vi "monitor_old.vi"() -> ()   [LabVIEW 2010]
uses:
  <vilib>/Instr/_visa.llb/VISA Configure Serial Port (Instr).vi
panel:
  out "start time":timestamp
  in  "Boolean 6":bool
  in  "Log file":path=path "C:/write-read example.txt"
  in  "Boolean 5":bool
  in  "Log file":path=path "C:/write-read example.txt"
  in  "Boolean 4":bool
  in  "Log file":path=path "C:/write-read example.txt"
  in  "Boolean 3":bool
  in  "Log file":path=path "C:/write-read example.txt"
  in  "Boolean 2":bool
  in  "Log file":path=path "C:/write-read example.txt"
  in  "Boolean":bool
  in  "Log file":path=path "C:/write-read example.txt"
  out "Power":dbl format="%.2g"
  out "Power":dbl format="%.2g"
  out "Power":dbl format="%.2g"
  out "Power":dbl format="%.2g"
  out "Power":dbl format="%.2g"
  out "Power":dbl format="%.2g"
  out "readPower":string=">\\s$R153\\?\\r\\n"
  in  "Connect all":bool
  out "Voltage":dbl format="%.2g"
  out "Current":dbl format="%.2g"
  out "Regulator":dbl format="%.2g"
  out "Extra sensor":dbl format="%.2g"
  out "Cold plate":dbl format="%.2g"
  out "Set point":dbl format="%.2g"
  out "Main sensor":dbl format="%.2g"
  out "Voltage":dbl format="%.2g"
  out "Current":dbl format="%.2g"
  out "Regulator":dbl format="%.2g"
  out "Extra sensor":dbl format="%.2g"
  out "Cold plate":dbl format="%.2g"
  out "Set point":dbl format="%.2g"
  out "Sensor":dbl format="%.2g"
  out "Voltage":dbl format="%.2g"
  out "Current":dbl format="%.2g"
  out "Regulator":dbl format="%.2g"
  out "Extra sensor":dbl format="%.2g"
  out "Cold plate":dbl format="%.2g"
  out "Set point":dbl format="%.2g"
  out "Main sensor":dbl format="%.2g"
  out "Voltage":dbl format="%.2g"
  out "Current":dbl format="%.2g"
  out "Regulator":dbl format="%.2g"
  out "Extra sensor":dbl format="%.2g"
  out "Cold plate":dbl format="%.2g"
  out "Set point":dbl format="%.2g"
  out "Sensor":dbl format="%.2g"
  out "Voltage":dbl format="%.2g"
  out "Current":dbl format="%.2g"
  out "Regulator":dbl format="%.2g"
  out "Extra sensor":dbl format="%.2g"
  out "Cold plate":dbl format="%.2g"
  out "Set point":dbl format="%.2g"
  out "Main sensor":dbl format="%.2g"
  out "readI":string=">\\s$R101\\?\\r\\n"
  out "readV":string=">\\s$R101\\?\\r\\n"
  out "readT4":string=">\\s$R101\\?\\r\\n"
  out "Voltage":dbl format="%.2g"
  out "Current":dbl format="%.2g"
  out "Regulator":dbl format="%.2g"
  out "readT3":string=">\\s$R101\\?\\r\\n"
  out "Extra sensor":dbl format="%.2g"
  out "Cold plate":dbl format="%.2g"
  out "Set point":dbl format="%.2g"
  out "readT2":string=">\\s$R101\\?\\r\\n"
  out "readT1":string=">\\s$R100\\?\\r\\n"
  out "readSetPoint":string="$R0\\?\\r\\n"
  out "Main sensor":dbl format="%.2g"
  in  "Port":refnum<visa-resource-name>="COM7"
  in  "Port":refnum<visa-resource-name>="COM6"
  in  "Port":refnum<visa-resource-name>="COM11"
  in  "Port":refnum<visa-resource-name>="COM10"
  in  "Port":refnum<visa-resource-name>="COM9"
  in  "Port":refnum<visa-resource-name>="COM8"
  in  "stop":bool
  # "Top S"
  # "Top N"
  # "Temeprature"
  # "Temeprature"
  # "Bottom S"
  # "Bottom N"
  # "Temeprature"
  # "Temeprature"
  # "Front S"
  # "Front N"
  # "Temeprature"
  # "Temeprature"
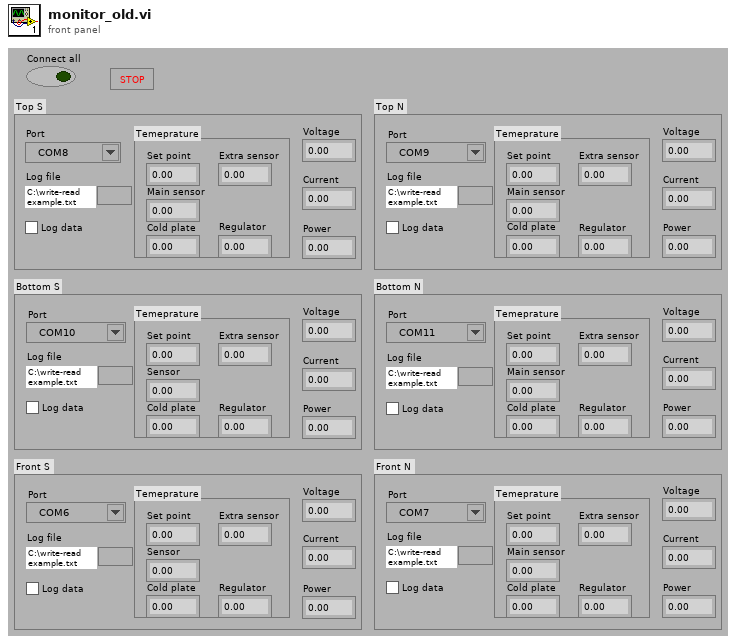
[diagram p1: front panel]
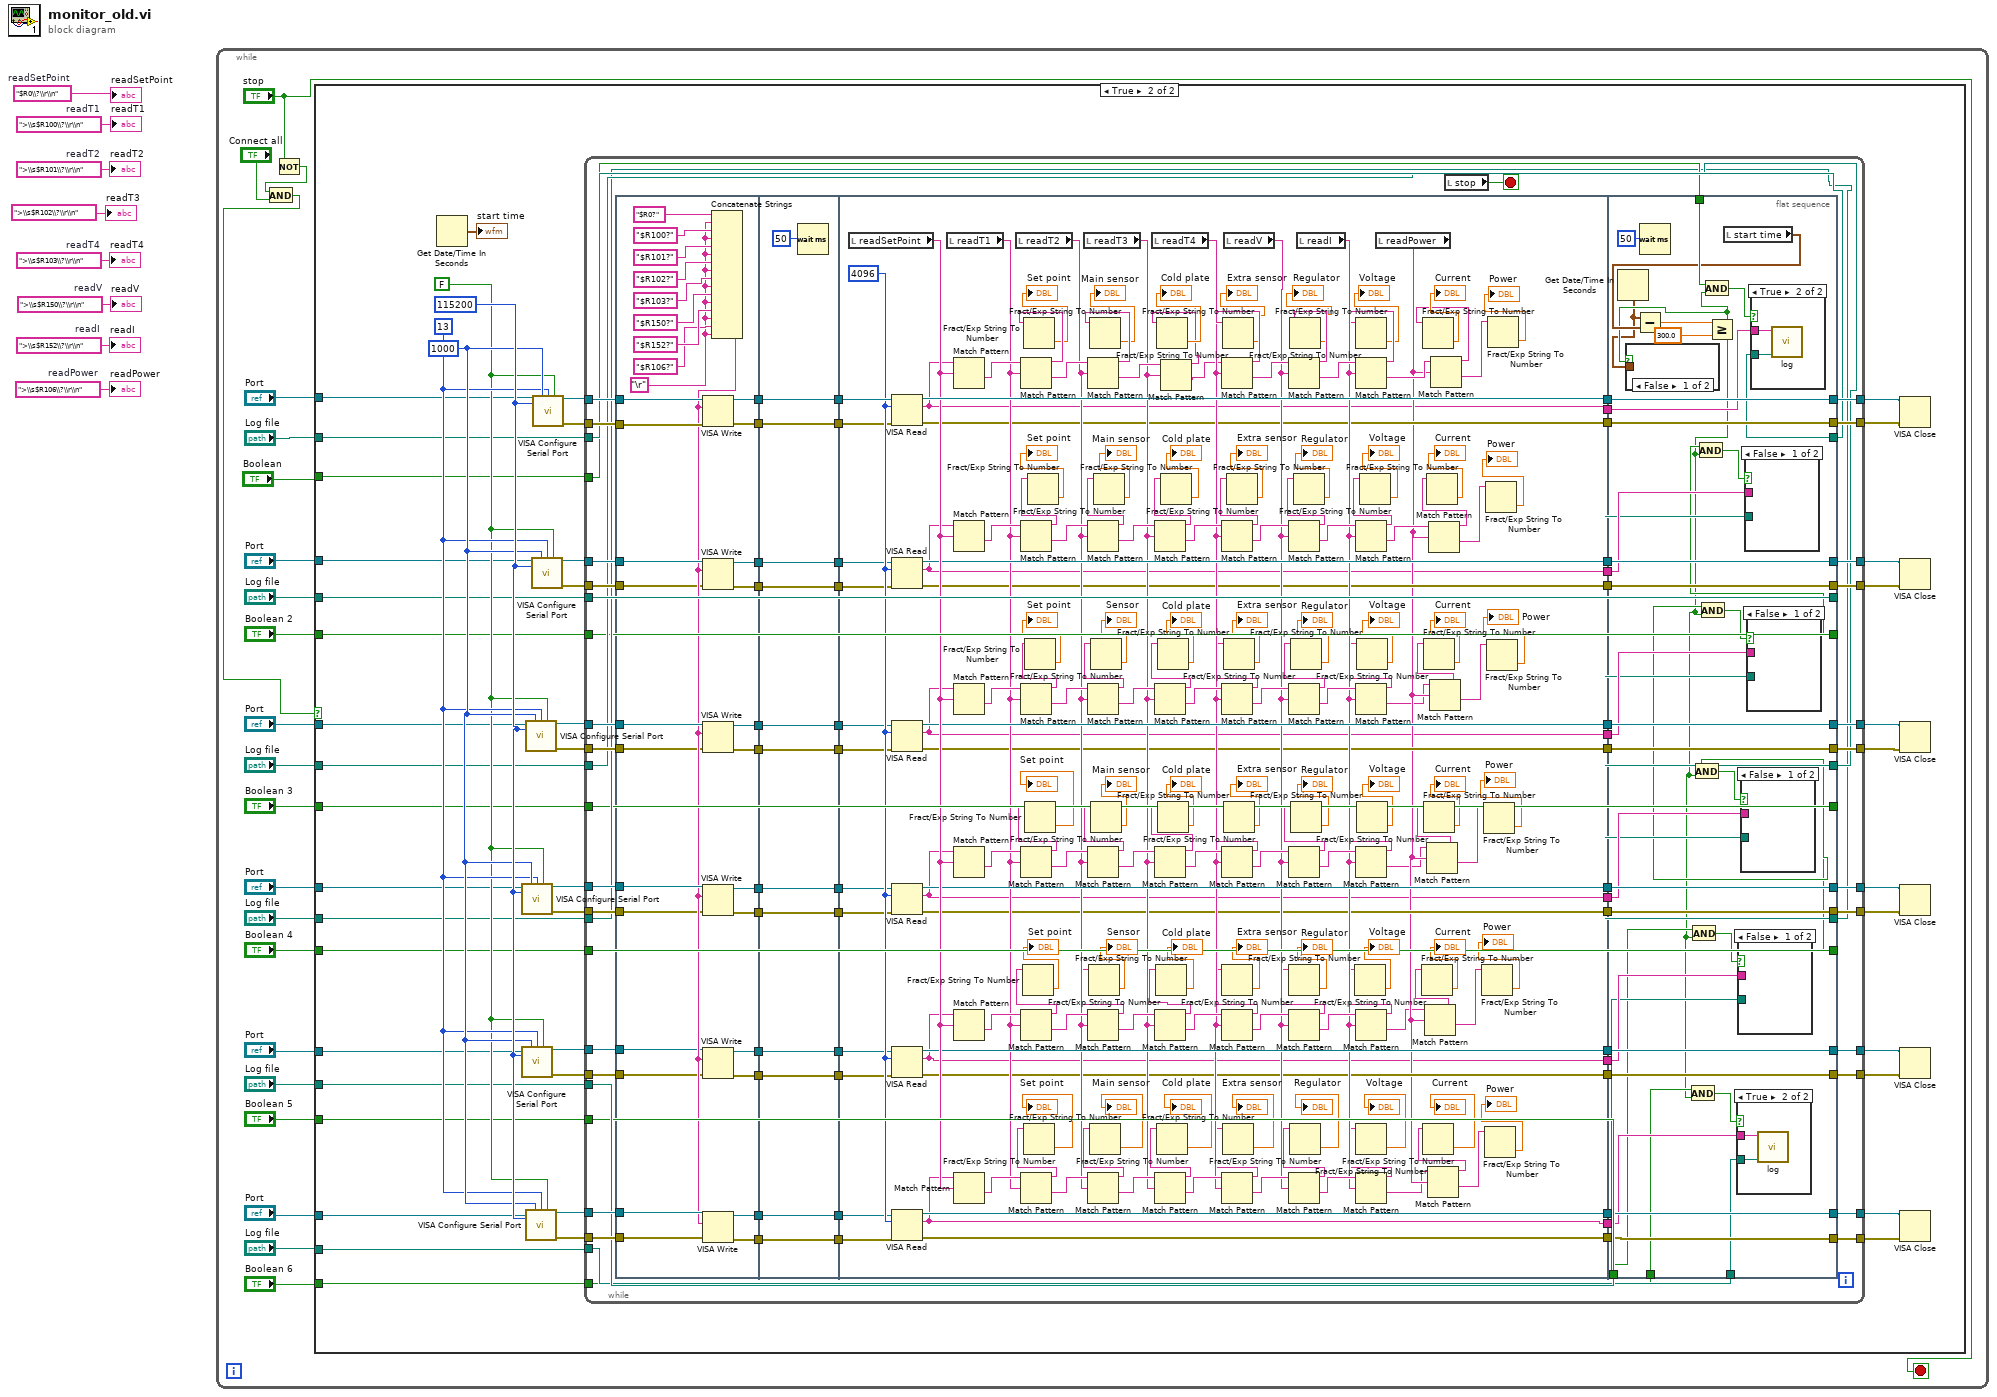
[diagram p0: block diagram]
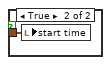
[diagram p3: hidden frame]
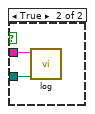
[diagram p5: hidden frame]
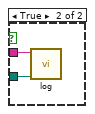
[diagram p6: hidden frame]
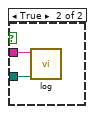
[diagram p7: hidden frame]
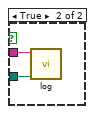
[diagram p8: hidden frame]
diagram:
  w1 = ">\\s$R106\\?\\r\\n"  # readPower
  w2 = ">\\s$R152\\?\\r\\n"  # readI
  w3 = ">\\s$R150\\?\\r\\n"  # readV
  w4 = ">\\s$R103\\?\\r\\n"  # readT4
  w6 = ">\\s$R101\\?\\r\\n"  # readT2
  w7 = ">\\s$R100\\?\\r\\n"  # readT1
  w8 = "$R0\\?\\r\\n"  # readSetPoint
  n1 = while {
    stop <- "stop" stop-if-true
    n2 = Not(x="stop") -> (.not. x?=w10:bool)
    n3 = And(x=w10, y="Connect all") -> (x .and. y?=w11:bool)
    n4 = case shown="True" w11 {
      tunnel: "Port" -> [_ w67]
      tunnel: "Port" -> [_ w66]
      tunnel: "Port" -> [_ w65]
      tunnel: "Port" -> [_ w64]
      tunnel: "Port" -> [_ w63]
      tunnel: "Port" -> [_ w62]
      tunnel: "Log file" -> [_ w55]
      tunnel: "Boolean" -> [_ w54]
      tunnel: "Log file" -> [_ w53]
      tunnel: "Log file" -> [_ w52]
      tunnel: "Log file" -> [_ w51]
      tunnel: "Log file" -> [_ w50]
      tunnel: "Log file" -> [_ w49]
      tunnel: "Boolean 2" -> [_ w48]
      tunnel: "Boolean 3" -> [_ w47]
      tunnel: "Boolean 4" -> [_ w46]
      tunnel: "Boolean 5" -> [_ w45]
      tunnel: "Boolean 6" -> [_ w44]
      frame False {
      }
      frame True {
        w71 = u32 115200 ("baud rate (9600)")
        w70 = u32 1000 ("timeout (10sec)")
        w68 = FALSE ("Enable Termination\nChar (T)")
        w69 = u8 13 ("termination char\n(0xA = '\\n' = LF)")
        n5 = Get Date/Time In Seconds() -> (seconds since 1Jan1904=→"start time":timestamp)
        n6 = call-poly "VISA Configure Serial Port"("VISA resource name"=w64, "timeout (10sec)"=w70, "termination char\n(0xA = '\\n' = LF)"=w69, "Enable Termination\nChar (T)"=w68, "baud rate (9600)"=w71) -> ("VISA resource name out"=w74:refnum<visa-resource-name>, "error out"=w57:errorcluster)  [unwired: 9 in]
        n7 = call-poly "VISA Configure Serial Port"("VISA resource name"=w63, "timeout (10sec)"=w70, "termination char\n(0xA = '\\n' = LF)"=w69, "Enable Termination\nChar (T)"=w68, "baud rate (9600)"=w71) -> ("VISA resource name out"=w73:refnum<visa-resource-name>, "error out"=w56:errorcluster)  [unwired: 9 in]
        n8 = call-poly "VISA Configure Serial Port"("VISA resource name"=w65, "timeout (10sec)"=w70, "termination char\n(0xA = '\\n' = LF)"=w69, "Enable Termination\nChar (T)"=w68, "baud rate (9600)"=w71) -> ("VISA resource name out"=w75:refnum<visa-resource-name>, "error out"=w58:errorcluster)  [unwired: 9 in]
        n9 = call-poly "VISA Configure Serial Port"("VISA resource name"=w62, "timeout (10sec)"=w70, "termination char\n(0xA = '\\n' = LF)"=w69, "Enable Termination\nChar (T)"=w68, "baud rate (9600)"=w71) -> ("VISA resource name out"=w72:refnum<visa-resource-name>, "error out"=w61:errorcluster)  [unwired: 9 in]
        n10 = call-poly "VISA Configure Serial Port"("VISA resource name"=w66, "timeout (10sec)"=w70, "termination char\n(0xA = '\\n' = LF)"=w69, "Enable Termination\nChar (T)"=w68, "baud rate (9600)"=w71) -> ("VISA resource name out"=w76:refnum<visa-resource-name>, "error out"=w59:errorcluster)  [unwired: 9 in]
        n11 = call-poly "VISA Configure Serial Port"("VISA resource name"=w67, "timeout (10sec)"=w70, "termination char\n(0xA = '\\n' = LF)"=w69, "Enable Termination\nChar (T)"=w68, "baud rate (9600)"=w71) -> ("VISA resource name out"=w77:refnum<visa-resource-name>, "error out"=w60:errorcluster)  [unwired: 9 in]
        n12 = while {
          tunnel: w77 -> [w153]
          tunnel: [w152] -> w42
          tunnel: w76 -> [w151]
          tunnel: w75 -> [w150]
          tunnel: w74 -> [w149]
          tunnel: w73 -> [w148]
          tunnel: w72 -> [w147]
          tunnel: [w143] -> w40
          tunnel: [w133] -> w34
          tunnel: [w130] -> w38
          tunnel: [w129] -> w36
          tunnel: [w127] -> w31
          tunnel: [w126] -> w32
          tunnel: w61 -> [w118]
          tunnel: w60 -> [w123]
          tunnel: w59 -> [w122]
          tunnel: w58 -> [w121]
          tunnel: w57 -> [w120]
          tunnel: w56 -> [w119]
          tunnel: [w105] -> w41
          tunnel: [w103] -> w39
          tunnel: [w101] -> w37
          tunnel: [w99] -> w35
          tunnel: [w97] -> w33
          tunnel: w55 -> [w95]
          tunnel: w54 -> [w94]
          tunnel: w53 -> [w88]
          tunnel: w52 -> [w87]
          tunnel: w51 -> [w86]
          tunnel: w50 -> [w85]
          tunnel: w49 -> [w84]
          tunnel: w48 -> [w83]
          tunnel: w47 -> [w82]
          tunnel: w46 -> [w81]
          tunnel: w45 -> [w80]
          tunnel: w44 -> [w79]
          stop <- w78 stop-if-true
          n13 = flat-sequence {
            tunnel: w153 -> [w190]
            tunnel: w123 -> [w188]
            tunnel: [w189] -> w156
            tunnel: w151 -> [w187]
            tunnel: w150 -> [w186]
            tunnel: w149 -> [w185]
            tunnel: w148 -> [w169]
            tunnel: w147 -> [w184]
            tunnel: [w183] -> w145
            tunnel: [w182] -> w141
            tunnel: [w181] -> w140
            tunnel: [w180] -> w138
            tunnel: [w179] -> w136
            tunnel: [w178] -> w134
            tunnel: w122 -> [w168]
            tunnel: w121 -> [w167]
            tunnel: w120 -> [w166]
            tunnel: w119 -> [w165]
            tunnel: w118 -> [w164]
            tunnel: [w163] -> w116
            tunnel: [w162] -> w114
            tunnel: [w161] -> w112
            tunnel: [w160] -> w110
            tunnel: [w159] -> w108
            tunnel: w156 -> [w203]
            tunnel: [w203] -> w155
            tunnel: [w201] -> w146
            tunnel: w145 -> [w201]
            tunnel: [w200] -> w142
            tunnel: w141 -> [w200]
            tunnel: w140 -> [w191]
            tunnel: [w199] -> w139
            tunnel: w138 -> [w199]
            tunnel: [w198] -> w137
            tunnel: w136 -> [w198]
            tunnel: [w197] -> w135
            tunnel: w134 -> [w197]
            tunnel: [w196] -> w117
            tunnel: w116 -> [w196]
            tunnel: [w195] -> w115
            tunnel: w114 -> [w195]
            tunnel: [w194] -> w113
            tunnel: w112 -> [w194]
            tunnel: [w193] -> w111
            tunnel: w110 -> [w193]
            tunnel: [w192] -> w109
            tunnel: w108 -> [w192]
            tunnel: [w191] -> w107
            tunnel: w155 -> [w380]
            tunnel: [w379] -> w154
            tunnel: w146 -> [w339]
            tunnel: [w337] -> w144
            tunnel: w142 -> [w341]
            tunnel: w139 -> [w342]
            tunnel: w137 -> [w340]
            tunnel: w135 -> [w343]
            tunnel: [w335] -> w132
            tunnel: [w336] -> w131
            tunnel: [w338] -> w128
            tunnel: [w334] -> w125
            tunnel: [w333] -> w124
            tunnel: w117 -> [w310]
            tunnel: w115 -> [w309]
            tunnel: w113 -> [w308]
            tunnel: w111 -> [w307]
            tunnel: w109 -> [w306]
            tunnel: w107 -> [w305]
            tunnel: [w304] -> w106
            tunnel: [w303] -> w104
            tunnel: [w302] -> w102
            tunnel: [w301] -> w100
            tunnel: [w300] -> w98
            tunnel: [w209] -> w96
            tunnel: [w208] -> w93
            tunnel: [w207] -> w92
            tunnel: [w206] -> w91
            tunnel: [w205] -> w90
            tunnel: [w204] -> w89
            tunnel: w154 -> [w421]
            tunnel: [w421] -> w152
            tunnel: w144 -> [w420]
            tunnel: [w420] -> w143
            tunnel: [w419] -> w133
            tunnel: w132 -> [w417]
            tunnel: w131 -> [w418]
            tunnel: [w418] -> w130
            tunnel: [w417] -> w129
            tunnel: w128 -> [w415]
            tunnel: [w416] -> w127
            tunnel: [w415] -> w126
            tunnel: w125 -> [w419]
            tunnel: w124 -> [w416]
            tunnel: w106 -> [w414]
            tunnel: [w414] -> w105
            tunnel: w104 -> [w413]
            tunnel: [w413] -> w103
            tunnel: w102 -> [w412]
            tunnel: [w412] -> w101
            tunnel: w100 -> [w411]
            tunnel: [w411] -> w99
            tunnel: w98 -> [w410]
            tunnel: [w410] -> w97
            tunnel: w96 -> [w407]
            tunnel: w95 -> [w405]
            tunnel: w94 -> [w406]
            tunnel: w93 -> [w398]
            tunnel: w92 -> [w397]
            tunnel: w91 -> [w396]
            tunnel: w90 -> [w395]
            tunnel: w89 -> [w394]
            tunnel: w88 -> [w393]
            tunnel: w87 -> [w392]
            tunnel: w86 -> [w391]
            tunnel: w85 -> [w390]
            tunnel: w84 -> [w389]
            tunnel: w83 -> [w388]
            tunnel: w82 -> [w387]
            tunnel: w81 -> [w386]
            tunnel: w80 -> [w385]
            tunnel: w79 -> [w384]
            frame #0 {
              w157 = "\r"
              n14 = Concatenate Strings("$R0?" ("command"), w157, "$R100?" ("command"), w157, "$R101?" ("command"), w157, "$R102?" ("command"), w157, "$R103?" ("command"), w157, "$R150?" ("command"), w157, "$R152?" ("command"), w157, "$R106?" ("command"), w157) -> (w170:string)
              n15 = VISA Write(VISA resource name=w190, write buffer=w170, error in (no error)=w188) -> (VISA resource name out=w189:refnum<visa-resource-name>, error out=w163:errorcluster)  [unwired: 1 out]
              n16 = VISA Write(VISA resource name=w187, write buffer=w170, error in (no error)=w168) -> (VISA resource name out=w183:refnum<visa-resource-name>, error out=w162:errorcluster)  [unwired: 1 out]
              n17 = VISA Write(VISA resource name=w186, write buffer=w170, error in (no error)=w167) -> (VISA resource name out=w178:refnum<visa-resource-name>, error out=w161:errorcluster)  [unwired: 1 out]
              n18 = VISA Write(VISA resource name=w185, write buffer=w170, error in (no error)=w166) -> (VISA resource name out=w179:refnum<visa-resource-name>, error out=w160:errorcluster)  [unwired: 1 out]
              n19 = VISA Write(VISA resource name=w169, write buffer=w170, error in (no error)=w165) -> (VISA resource name out=w180:refnum<visa-resource-name>, error out=w159:errorcluster)  [unwired: 1 out]
              n20 = VISA Write(VISA resource name=w184, write buffer=w170, error in (no error)=w164) -> (VISA resource name out=w182:refnum<visa-resource-name>, error out=w181:errorcluster)  [unwired: 1 out]
            }
            frame #1 {
              n21 = Wait (ms)(milliseconds to wait=u32 50 ("attente (ms)")) -> ()  [unwired: 1 out]
            }
            frame #2 {
              w345 = u32 4096 ("nombre d'octets")
              n22 = local read "readSetPoint"() -> (w344:string)
              n23 = VISA Read(VISA resource name=w380, byte count=w345, error in (no error)=w310) -> (VISA resource name out=w379:refnum<visa-resource-name>, read buffer=w209:string, error out=w304:errorcluster)  [unwired: 1 out]
              n24 = VISA Read(VISA resource name=w339, byte count=w345, error in (no error)=w309) -> (VISA resource name out=w337:refnum<visa-resource-name>, read buffer=w208:string, error out=w303:errorcluster)  [unwired: 1 out]
              n25 = VISA Read(VISA resource name=w343, byte count=w345, error in (no error)=w308) -> (VISA resource name out=w336:refnum<visa-resource-name>, read buffer=w207:string, error out=w302:errorcluster)  [unwired: 1 out]
              n26 = VISA Read(VISA resource name=w340, byte count=w345, error in (no error)=w307) -> (VISA resource name out=w335:refnum<visa-resource-name>, read buffer=w206:string, error out=w301:errorcluster)  [unwired: 1 out]
              n27 = VISA Read(VISA resource name=w342, byte count=w345, error in (no error)=w306) -> (VISA resource name out=w334:refnum<visa-resource-name>, read buffer=w205:string, error out=w300:errorcluster)  [unwired: 1 out]
              n28 = VISA Read(VISA resource name=w341, byte count=w345, error in (no error)=w305) -> (VISA resource name out=w338:refnum<visa-resource-name>, read buffer=w204:string, error out=w333:errorcluster)  [unwired: 1 out]
              n29 = local read "readT1"() -> (w332:string)
              n30 = Match Pattern(string=w209, regular expression=w344) -> (after substring=w377:string)  [unwired: 1 in, 3 out]
              n31 = Match Pattern(string=w208, regular expression=w344) -> (after substring=w374:string)  [unwired: 1 in, 3 out]
              n32 = Match Pattern(string=w207, regular expression=w344) -> (after substring=w368:string)  [unwired: 1 in, 3 out]
              n33 = Match Pattern(string=w206, regular expression=w344) -> (after substring=w362:string)  [unwired: 1 in, 3 out]
              n34 = Match Pattern(string=w205, regular expression=w344) -> (after substring=w356:string)  [unwired: 1 in, 3 out]
              n35 = Match Pattern(string=w204, regular expression=w344) -> (after substring=w350:string)  [unwired: 1 in, 3 out]
              n36 = local read "readT2"() -> (w331:string)
              n37 = Match Pattern(string=w377, regular expression=w332) -> (before substring=w328:string, after substring=w378:string)  [unwired: 1 in, 2 out]
              n38 = Match Pattern(string=w374, regular expression=w332) -> (before substring=w299:string, after substring=w375:string)  [unwired: 1 in, 2 out]
              n39 = Match Pattern(string=w368, regular expression=w332) -> (before substring=w286:string, after substring=w369:string)  [unwired: 1 in, 2 out]
              n40 = Match Pattern(string=w362, regular expression=w332) -> (before substring=w267:string, after substring=w363:string)  [unwired: 1 in, 2 out]
              n41 = Match Pattern(string=w356, regular expression=w332) -> (before substring=w254:string, after substring=w357:string)  [unwired: 1 in, 2 out]
              n42 = Match Pattern(string=w350, regular expression=w332) -> (before substring=w247:string, after substring=w351:string)  [unwired: 1 in, 2 out]
              n43 = Fract/Exp String To Number(string=w254) -> (number=→"Set point":dbl)  [unwired: 3 in, 1 out]
              n44 = Fract/Exp String To Number(string=w328) -> (number=→"Set point":dbl)  [unwired: 3 in, 1 out]
              n45 = Fract/Exp String To Number(string=w247) -> (number=→"Set point":dbl)  [unwired: 3 in, 1 out]
              n46 = Fract/Exp String To Number(string=w286) -> (number=→"Set point":dbl)  [unwired: 3 in, 1 out]
              n47 = Fract/Exp String To Number(string=w267) -> (number=→"Set point":dbl)  [unwired: 3 in, 1 out]
              n48 = Fract/Exp String To Number(string=w299) -> (number=→"Set point":dbl)  [unwired: 3 in, 1 out]
              n49 = local read "readT3"() -> (w313:string)
              n50 = Match Pattern(string=w378, regular expression=w331) -> (before substring=w327:string, after substring=w314:string)  [unwired: 1 in, 2 out]
              n51 = Match Pattern(string=w375, regular expression=w331) -> (before substring=w298:string, after substring=w373:string)  [unwired: 1 in, 2 out]
              n52 = Match Pattern(string=w369, regular expression=w331) -> (before substring=w285:string, after substring=w367:string)  [unwired: 1 in, 2 out]
              n53 = Match Pattern(string=w363, regular expression=w331) -> (before substring=w273:string, after substring=w361:string)  [unwired: 1 in, 2 out]
              n54 = Match Pattern(string=w357, regular expression=w331) -> (before substring=w255:string, after substring=w355:string)  [unwired: 1 in, 2 out]
              n55 = Match Pattern(string=w351, regular expression=w331) -> (before substring=w246:string, after substring=w349:string)  [unwired: 1 in, 2 out]
              n56 = Fract/Exp String To Number(string=w255) -> (number=→"Sensor":dbl)  [unwired: 3 in, 1 out]
              n57 = Fract/Exp String To Number(string=w327) -> (number=→"Main sensor":dbl)  [unwired: 3 in, 1 out]
              n58 = Fract/Exp String To Number(string=w246) -> (number=→"Main sensor":dbl)  [unwired: 3 in, 1 out]
              n59 = Fract/Exp String To Number(string=w285) -> (number=→"Sensor":dbl)  [unwired: 3 in, 1 out]
              n60 = Fract/Exp String To Number(string=w273) -> (number=→"Main sensor":dbl)  [unwired: 3 in, 1 out]
              n61 = Fract/Exp String To Number(string=w298) -> (number=→"Main sensor":dbl)  [unwired: 3 in, 1 out]
              n62 = local read "readT4"() -> (w315:string)
              n63 = Match Pattern(string=w373, regular expression=w313) -> (before substring=w297:string, after substring=w372:string)  [unwired: 1 in, 2 out]
              n64 = Match Pattern(string=w367, regular expression=w313) -> (before substring=w284:string, after substring=w366:string)  [unwired: 1 in, 2 out]
              n65 = Match Pattern(string=w361, regular expression=w313) -> (before substring=w272:string, after substring=w360:string)  [unwired: 1 in, 2 out]
              n66 = Match Pattern(string=w355, regular expression=w313) -> (before substring=w256:string, after substring=w354:string)  [unwired: 1 in, 2 out]
              n67 = Match Pattern(string=w349, regular expression=w313) -> (before substring=w245:string, after substring=w348:string)  [unwired: 1 in, 2 out]
              n68 = Fract/Exp String To Number(string=w256) -> (number=→"Cold plate":dbl)  [unwired: 3 in, 1 out]
              n69 = Fract/Exp String To Number(string=w245) -> (number=→"Cold plate":dbl)  [unwired: 3 in, 1 out]
              n70 = Fract/Exp String To Number(string=w284) -> (number=→"Cold plate":dbl)  [unwired: 3 in, 1 out]
              n71 = Fract/Exp String To Number(string=w272) -> (number=→"Cold plate":dbl)  [unwired: 3 in, 1 out]
              n72 = Match Pattern(string=w314, regular expression=w313) -> (before substring=w312:string, after substring=w311:string)  [unwired: 1 in, 2 out]
              n73 = Fract/Exp String To Number(string=w312) -> (number=→"Cold plate":dbl)  [unwired: 3 in, 1 out]
              n74 = Fract/Exp String To Number(string=w297) -> (number=→"Cold plate":dbl)  [unwired: 3 in, 1 out]
              n75 = Match Pattern(string=w311, regular expression=w315) -> (before substring=w326:string, after substring=w317:string)  [unwired: 1 in, 2 out]
              n76 = Match Pattern(string=w372, regular expression=w315) -> (before substring=w296:string, after substring=w371:string)  [unwired: 1 in, 2 out]
              n77 = Match Pattern(string=w366, regular expression=w315) -> (before substring=w283:string, after substring=w365:string)  [unwired: 1 in, 2 out]
              n78 = Match Pattern(string=w360, regular expression=w315) -> (before substring=w271:string, after substring=w359:string)  [unwired: 1 in, 2 out]
              n79 = Match Pattern(string=w354, regular expression=w315) -> (before substring=w257:string, after substring=w353:string)  [unwired: 1 in, 2 out]
              n80 = Fract/Exp String To Number(string=w257) -> (number=→"Extra sensor":dbl)  [unwired: 3 in, 1 out]
              n81 = Match Pattern(string=w348, regular expression=w315) -> (before substring=w244:string, after substring=w347:string)  [unwired: 1 in, 2 out]
              n82 = Fract/Exp String To Number(string=w326) -> (number=→"Extra sensor":dbl)  [unwired: 3 in, 1 out]
              n83 = Fract/Exp String To Number(string=w244) -> (number=→"Extra sensor":dbl)  [unwired: 3 in, 1 out]
              n84 = local read "readV"() -> (w316:string)
              n85 = Fract/Exp String To Number(string=w283) -> (number=→"Extra sensor":dbl)  [unwired: 3 in, 1 out]
              n86 = Fract/Exp String To Number(string=w271) -> (number=→"Extra sensor":dbl)  [unwired: 3 in, 1 out]
              n87 = Fract/Exp String To Number(string=w296) -> (number=→"Extra sensor":dbl)  [unwired: 3 in, 1 out]
              n88 = Match Pattern(string=w317, regular expression=w316) -> (before substring=w325:string, after substring=w376:string)  [unwired: 1 in, 2 out]
              n89 = Match Pattern(string=w371, regular expression=w316) -> (before substring=w295:string, after substring=w370:string)  [unwired: 1 in, 2 out]
              n90 = Match Pattern(string=w365, regular expression=w316) -> (before substring=w282:string, after substring=w364:string)  [unwired: 1 in, 2 out]
              n91 = Match Pattern(string=w359, regular expression=w316) -> (before substring=w270:string, after substring=w358:string)  [unwired: 1 in, 2 out]
              n92 = Match Pattern(string=w353, regular expression=w316) -> (before substring=w258:string, after substring=w352:string)  [unwired: 1 in, 2 out]
              n93 = Fract/Exp String To Number(string=w258) -> (number=→"Regulator":dbl)  [unwired: 3 in, 1 out]
              n94 = Match Pattern(string=w347, regular expression=w316) -> (before substring=w243:string, after substring=w346:string)  [unwired: 1 in, 2 out]
              n95 = Fract/Exp String To Number(string=w325) -> (number=→"Regulator":dbl)  [unwired: 3 in, 1 out]
              n96 = Fract/Exp String To Number(string=w243) -> (number=→"Regulator":dbl)  [unwired: 3 in, 1 out]
              n97 = Fract/Exp String To Number(string=w282) -> (number=→"Regulator":dbl)  [unwired: 3 in, 1 out]
              n98 = Fract/Exp String To Number(string=w270) -> (number=→"Regulator":dbl)  [unwired: 3 in, 1 out]
              n99 = Fract/Exp String To Number(string=w295) -> (number=→"Regulator":dbl)  [unwired: 3 in, 1 out]
              n100 = local read "readI"() -> (w330:string)
              n101 = Match Pattern(string=w376, regular expression=w330) -> (before substring=w324:string, after substring=w234:string)  [unwired: 1 in, 2 out]
              n102 = Fract/Exp String To Number(string=w324) -> (number=→"Voltage":dbl)  [unwired: 3 in, 1 out]
              n103 = Match Pattern(string=w370, regular expression=w330) -> (before substring=w294:string, after substring=w220:string)  [unwired: 1 in, 2 out]
              n104 = Match Pattern(string=w364, regular expression=w330) -> (before substring=w281:string, after substring=w217:string)  [unwired: 1 in, 2 out]
              n105 = Match Pattern(string=w358, regular expression=w330) -> (before substring=w269:string, after substring=w216:string)  [unwired: 1 in, 2 out]
              n106 = Match Pattern(string=w352, regular expression=w330) -> (before substring=w259:string, after substring=w212:string)  [unwired: 1 in, 2 out]
              n107 = Fract/Exp String To Number(string=w259) -> (number=→"Voltage":dbl)  [unwired: 3 in, 1 out]
              n108 = Match Pattern(string=w346, regular expression=w330) -> (before substring=w242:string, after substring=w211:string)  [unwired: 1 in, 2 out]
              n109 = Fract/Exp String To Number(string=w242) -> (number=→"Voltage":dbl)  [unwired: 3 in, 1 out]
              n110 = Fract/Exp String To Number(string=w281) -> (number=→"Voltage":dbl)  [unwired: 3 in, 1 out]
              n111 = Fract/Exp String To Number(string=w269) -> (number=→"Voltage":dbl)  [unwired: 3 in, 1 out]
              n112 = Fract/Exp String To Number(string=w294) -> (number=→"Voltage":dbl)  [unwired: 3 in, 1 out]
              n113 = local read "readPower"() -> (w218:string)
              n114 = Match Pattern(string=w212, regular expression=w218) -> (before substring=w213:string, after substring=w224:string)  [unwired: 1 in, 2 out]
              n115 = Fract/Exp String To Number(string=w213) -> (number=→"Current":dbl)  [unwired: 3 in, 1 out]
              n116 = Match Pattern(string=w216, regular expression=w218) -> (before substring=w214:string, after substring=w226:string)  [unwired: 1 in, 2 out]
              n117 = Fract/Exp String To Number(string=w214) -> (number=→"Current":dbl)  [unwired: 3 in, 1 out]
              n118 = Match Pattern(string=w211, regular expression=w218) -> (before substring=w210:string, after substring=w222:string)  [unwired: 1 in, 2 out]
              n119 = Fract/Exp String To Number(string=w210) -> (number=→"Current":dbl)  [unwired: 3 in, 1 out]
              n120 = Match Pattern(string=w220, regular expression=w218) -> (before substring=w219:string, after substring=w230:string)  [unwired: 1 in, 2 out]
              n121 = Fract/Exp String To Number(string=w219) -> (number=→"Current":dbl)  [unwired: 3 in, 1 out]
              n122 = Match Pattern(string=w217, regular expression=w218) -> (before substring=w215:string, after substring=w228:string)  [unwired: 1 in, 2 out]
              n123 = Fract/Exp String To Number(string=w215) -> (number=→"Current":dbl)  [unwired: 3 in, 1 out]
              n124 = Match Pattern(string=w234, regular expression=w218) -> (before substring=w233:string, after substring=w232:string)  [unwired: 1 in, 2 out]
              n125 = Fract/Exp String To Number(string=w233) -> (number=→"Current":dbl)  [unwired: 3 in, 1 out]
              n126 = Fract/Exp String To Number(string=w224) -> (number=→"Power":dbl)  [unwired: 3 in, 1 out]
              n127 = Fract/Exp String To Number(string=w226) -> (number=→"Power":dbl)  [unwired: 3 in, 1 out]
              n128 = Fract/Exp String To Number(string=w222) -> (number=→"Power":dbl)  [unwired: 3 in, 1 out]
              n129 = Fract/Exp String To Number(string=w230) -> (number=→"Power":dbl)  [unwired: 3 in, 1 out]
              n130 = Fract/Exp String To Number(string=w228) -> (number=→"Power":dbl)  [unwired: 3 in, 1 out]
              n131 = Fract/Exp String To Number(string=w232) -> (number=→"Power":dbl)  [unwired: 3 in, 1 out]
            }
            frame #3 {
              n132 = Get Date/Time In Seconds() -> (seconds since 1Jan1904=w381:timestamp)
              n133 = Wait (ms)(milliseconds to wait=u32 50 ("attente (ms)")) -> ()  [unwired: 1 out]
              n134 = local read "start time"() -> (w383:timestamp)
              n135 = Subtract(x=w381, y=w383) -> (x-y=w404:dbl)
              n136 = Greater Or Equal?(x=w404, y=300.0) -> (x >= y?=w382:bool)
              n137 = case shown="False" w382 {
                tunnel: w381 -> [_ w423]
                frame False {
                }
                frame True {
                  n138 = local write "start time"(w423) -> ()
                }
              }
              n139 = And(x=w384, y=w382) -> (x .and. y?=w399:bool)
              n140 = And(x=w385, y=w382) -> (x .and. y?=w400:bool)
              n141 = And(x=w386, y=w382) -> (x .and. y?=w401:bool)
              n142 = And(x=w388, y=w382) -> (x .and. y?=w403:bool)
              n143 = And(x=w387, y=w382) -> (x .and. y?=w402:bool)
              n144 = And(x=w406, y=w382) -> (x .and. y?=w408:bool)
              n145 = case shown="True" w399 {
                tunnel: w389 -> [_ w425]
                tunnel: w394 -> [_ w424]
                frame False {
                }
                frame True {
                  n146 = call "log.vi"("error in (no error)"=w425, "Data"=w424) -> ()  [unwired: 8 in, 2 out]
                }
              }
              n147 = case shown="False" w400 {
                tunnel: w390 -> [_ w427]
                tunnel: w395 -> [_ w426]
                frame False {
                }
                frame True {
                  n148 = call "log.vi"("error in (no error)"=w427, "Data"=w426) -> ()  [unwired: 8 in, 2 out]
                }
              }
              n149 = case shown="False" w401 {
                tunnel: w391 -> [_ w429]
                tunnel: w396 -> [_ w428]
                frame False {
                }
                frame True {
                  n150 = call "log.vi"("error in (no error)"=w429, "Data"=w428) -> ()  [unwired: 8 in, 2 out]
                }
              }
              n151 = case shown="False" w403 {
                tunnel: w393 -> [_ w433]
                tunnel: w398 -> [_ w432]
                frame False {
                }
                frame True {
                  n152 = call "log.vi"("error in (no error)"=w433, "Data"=w432) -> ()  [unwired: 8 in, 2 out]
                }
              }
              n153 = case shown="False" w402 {
                tunnel: w392 -> [_ w431]
                tunnel: w397 -> [_ w430]
                frame False {
                }
                frame True {
                  n154 = call "log.vi"("error in (no error)"=w431, "Data"=w430) -> ()  [unwired: 8 in, 2 out]
                }
              }
              n155 = case shown="True" w408 {
                tunnel: w405 -> [_ w435]
                tunnel: w407 -> [_ w434]
                frame False {
                }
                frame True {
                  n156 = call "log.vi"("error in (no error)"=w435, "Data"=w434) -> ()  [unwired: 8 in, 2 out]
                }
              }
            }
          }
          n157 = local read "stop"() -> (w78:bool)
        }
        n158 = VISA Close(VISA resource name=w42, error in (no error)=w41) -> ()  [unwired: 1 out]
        n159 = VISA Close(VISA resource name=w40, error in (no error)=w39) -> ()  [unwired: 1 out]
        n160 = VISA Close(VISA resource name=w38, error in (no error)=w37) -> ()  [unwired: 1 out]
        n161 = VISA Close(VISA resource name=w36, error in (no error)=w35) -> ()  [unwired: 1 out]
        n162 = VISA Close(VISA resource name=w34, error in (no error)=w33) -> ()  [unwired: 1 out]
        n163 = VISA Close(VISA resource name=w32, error in (no error)=w31) -> ()  [unwired: 1 out]
      }
    }
  }
  "readSetPoint" <- w8
  "readT1" <- w7
  "readT2" <- w6
  "readT3" <- ">\\s$R102\\?\\r\\n" ("readT3 2")
  "readT4" <- w4
  "readV" <- w3
  "readI" <- w2
  "readPower" <- w1
